vi "promptSaveNodes.vi"(8 "error in (no error)":errorcluster, 11 "xceRootNode in":refnum<class "xceRootNode.lvclass">) -> (0 "error out":errorcluster, 1 "cancelled":bool, 3 "xceRootNode out":refnum<class "xceRootNode.lvclass">)   [LabVIEW 2013, in "xceRootNode.lvclass"]
doc: "Prompts the user if they would like to save the current configuration. The path they choose is stored in the xceRootNode for later use."
uses:
  xceRootNode.lvclass
  xceRootNode.lvclass/xceRootNode.ctl
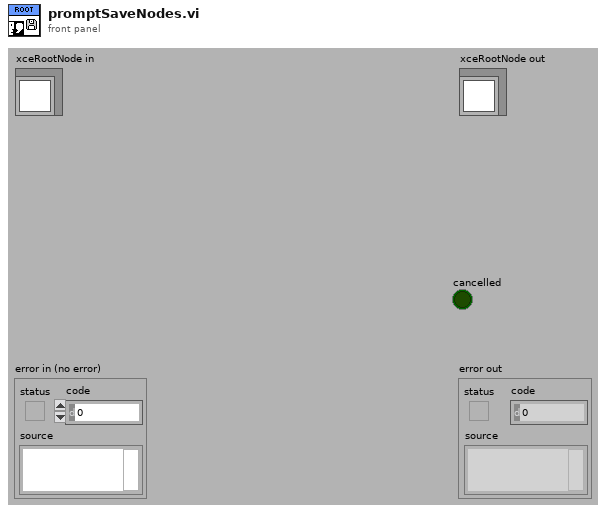
[diagram p1: front panel]
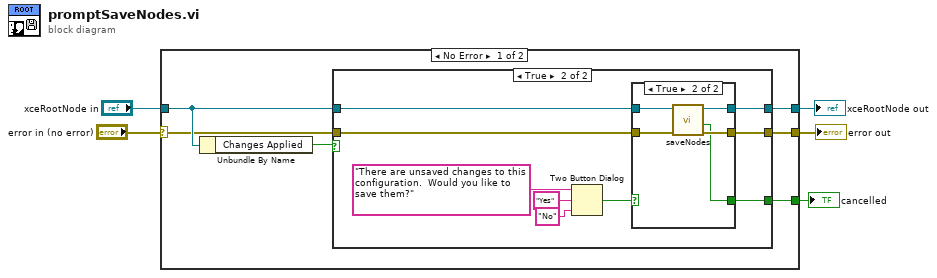
[diagram p0: block diagram]
diagram:
  n1 = case shown="No Error" "error in (no error)" {
    selector: "error in (no error)" -> [w8 w31]
    tunnel: [w7 w31] -> w4
    tunnel: [w9 w30] -> w2
    tunnel: "xceRootNode in" -> [w10 w30]
    tunnel: [w6 _] -> w1
    frame No Error {
      n2 = Unbundle By Name(w10) -> ("Changes Applied"=w11:bool)
      n3 = case shown="True" w11 {
        tunnel: w10 -> [w13 w19]
        tunnel: [w13 w18] -> w9
        tunnel: w8 -> [w12 w16]
        tunnel: [w12 w15] -> w7
        tunnel: [_ w14] -> w6
        frame False {
        }
        frame True {
          n4 = Two Button Dialog(message="There are unsaved changes to this configuration.  Would you like to save them?", 1:"No" ("F button name (\"Cancel\")"), 2:"Yes" ("T button name (\"OK\")")) -> (T button?=w17:bool)
          n5 = case shown="True" w17 {
            tunnel: w19 -> [w24 w29]
            tunnel: [w24 w28] -> w18
            tunnel: w16 -> [w23 w27]
            tunnel: [w23 w26] -> w15
            tunnel: [_ w25] -> w14
            frame False {
            }
            frame True {
              n6 = call "saveNodes.vi"("error in (no error)"=w27, "xceRootNode in"=w29) -> ("error out"=w26:errorcluster, "cancelled"=w25:bool, "xceRootNode out"=w28:refnum<class "xceRootNode.lvclass">)  [unwired: 7 in]
            }
          }
        }
      }
    }
    frame Error {
    }
  }
  "error out" <- w4
  "xceRootNode out" <- w2
  "cancelled" <- w1
